vi "Edit_ASCI_file.vi"() -> ()   [LabVIEW 2011]
panel:
  in  "start of read offset (chars.: 0)":i32
  in  "append to file? (new file:F)":bool
  in  "Mode":enum16{"Read", "Write"}(ring)
  in  "character string":string
  in  "file path (dialog if empty)":path
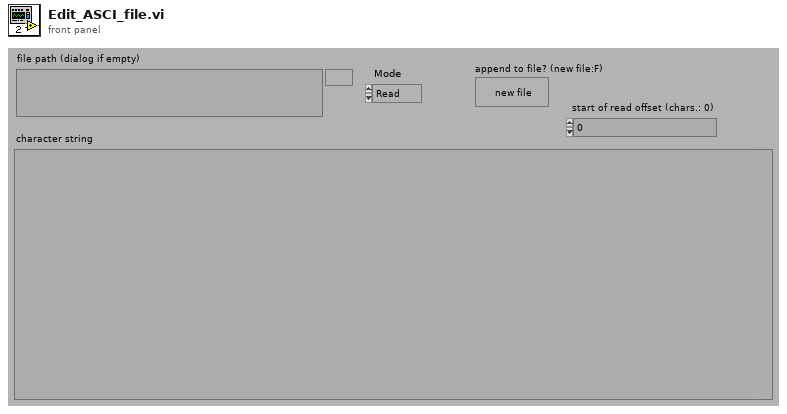
[diagram p1: front panel]
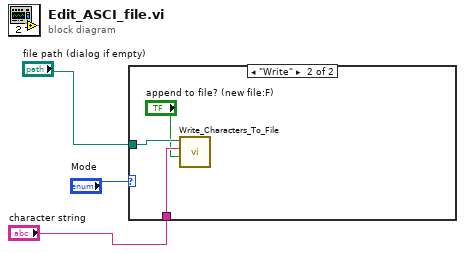
[diagram p0: block diagram]
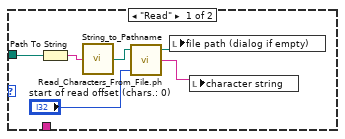
[diagram p2: hidden frame]
diagram:
  n1 = case shown="\"Write\"" "Mode" {
    tunnel: "file path (dialog if empty)" -> [w7 w12]
    tunnel: "character string" -> [_ w11]
    frame "Read" {
      n2 = Path To String(path=w7) -> (string=w6:string)
      n3 = call "String_to_Pathname.vi"("Input String"=w6) -> ("path"=w5:path)
      n4 = call "Read_Characters_From_File.ph.vi"("file path (dialog if empty)"=w5, "start of read offset (chars.: 0)"="start of read offset (chars.: 0)") -> ("new file path (NotAPath if cancelled)"=w9:path, "character string"=w8:string)  [unwired: 1 in, 5 out]
      n5 = local write "file path (dialog if empty)"(w9) -> ()
      n6 = local write "character string"(w8) -> ()
    }
    frame "Write" {
      n7 = call "Write_Characters_To_File.vi"("file path (dialog if empty)"=w12, "character string"=w11, "append to file? (new file:F)"="append to file? (new file:F)") -> ()  [unwired: 2 in, 4 out]
    }
  }
